vi "3.7-Reliable UDP Server Template.vi"() -> ()   [LabVIEW 2010]
doc: "UDP Mutlicast Addressing Scheme:\n\n3.7 - Multicast Address: 133.7.3.7\n3.1-4.7.1 Port: 31471\n3.2-4.7.2 Port: 32472\n3.3-4.7.3 Port: 33473\n3.4-4.7.4 Port: 34474\n\n5.7 - Multicast Address: 133.7.5.7\n5.1-4.7.1 Port: 51471\n5.2-4.7.2 Port: 52472\n5.3-4.7.3 Port: 53473\n5.4-4.7.4 Port: 54474\n\n5.1-6.7.1 Port: 51671\n5.2-6.7.2 Port: 52672\n5.3-6.7.3 Port: 53673\n5.4-6.7.4 Port: 54674\n\n7.7 - Multicast Address: 133.7.7.7\n7.1-6.7.1 Port: 61671\n7.2-6.7.2 Port: 62672\n7.3-6.7.3 Port: 63673\n7.4-6.7.4 Port: 64674"
uses:
  4-High Neurons/4.0-Super Heart Beat.ctl
  <vilib>/Utility/tcp.llb/UDP Multicast Write-Only Open.vi
  3.0-Global.vi
panel:
  out "Error":errorcluster
  in  "stop":bool
  out "Super Heart Beat":T1
  out "Processed":string
  in  "Debug Data":string
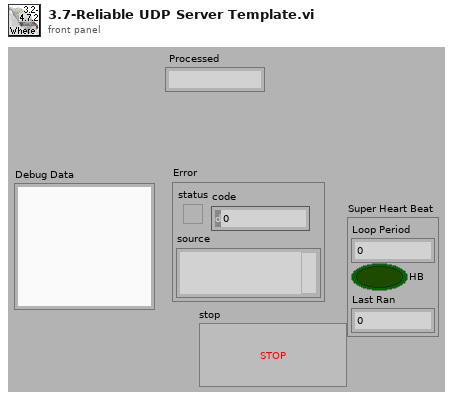
[diagram p1: front panel]
types:
  T1 = typedef "4.0-Super Heart Beat.ctl" = cluster{"Loop Period":u32, "HB":bool, "Last Ran":u32}
  T2 = typedef "3.3-What Sensor Typedef.ctl" = cluster{"LIDAR Data":T3}
  T3 = typedef "3.3.1-LIDAR Data Typedef.ctl" = cluster{"Angle array":dbl[], "Magnitude array ":dbl[]}
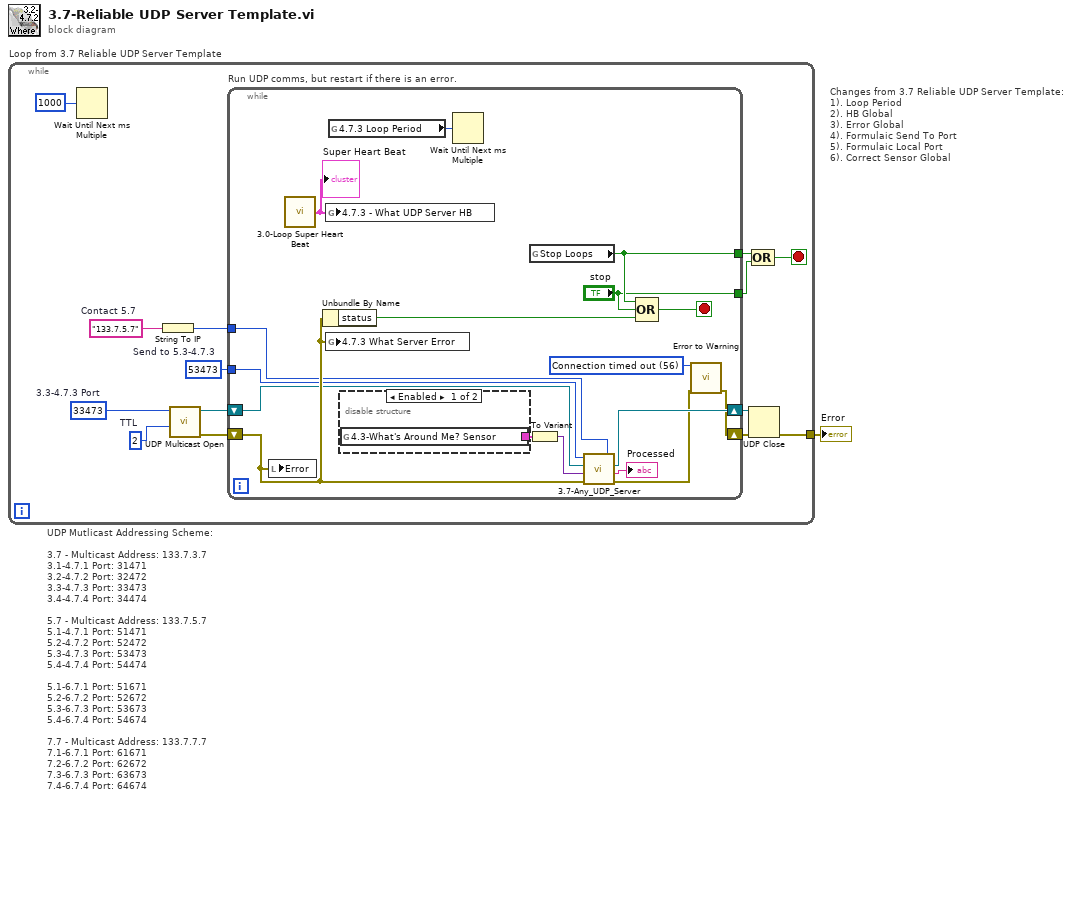
[diagram p0: block diagram]
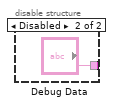
[diagram p2: hidden frame]
diagram:
  # "Changes from 3.7 Reliable UDP Server Template:\n1). Loop Period\n2). HB Global\n3). Error Global\n4). Formulaic Send To Port\n5). Formulaic Local Port\n6). Correct Sensor Global"
  # "UDP Mutlicast Addressing Scheme:\n\n3.7 - Multicast Address: 133.7.3.7\n3.1-4.7.1 Port: 31471\n3.2-4.7.2 Port: 32472\n3.3-4.7.3 Port: 33473\n3.4-4.7.4 Port: 34474\n\n5.7 - Multicast Address: 133.7.5.7\n5.1-4.7.1 Port: 51471\n5.2-4.7.2 Port: 52472\n5.3-4.7.3 Port: 53473\n5.4-4.7.4 Port: 54474\n\n5.1-6.7.1 Port: 51671\n5.2-6.7.2 Port: 52672\n5.3-6.7.3 Port: 53673\n5.4-6.7.4 Port: 54674\n\n7.7 - Multicast Address: 133.7.7.7\n7.1-6.7.1 Port: 61671\n7.2-6.7.2 Port: 62672\n7.3-6.7.3 Port: 63673\n7.4-6.7.4 Port: 64674"
  n1 = while "Loop from 3.7 Reliable UDP Server Template" {
    tunnel: [w10] -> w1
    stop <- w13 stop-if-true
    w2 = "133.7.5.7"  # Contact 5.7
    w4 = u16 53473  # Send to 5.3-4.7.3
    w7 = u16 2  # TTL
    w8 = u16 33473  # 3.3-4.7.3 Port
    n2 = Wait Until Next ms Multiple(millisecond multiple=u32 1000) -> ()  [unwired: 1 out]
    n3 = String To IP(1:w2) -> (0:w3:u32)
    n4 = call-poly <vilib>:"UDP Multicast Open.vi"("time-to-live (1)"=w7, "port"=w8) -> ("error out"=w5:errorcluster, "connection ID"=w6:refnum<k16>)  [unwired: 8 in]
    n5 = while "Run UDP comms, but restart if there is an error." {
      tunnel: [w31] -> w15
      tunnel: ["stop"] -> w14
      shift-right: [w22] -> w12
      shift-left: w6 -> [w23]
      shift-right: [w17] -> w11
      shift-left: w5 -> [w27]
      tunnel: w4 -> [w21]
      tunnel: w3 -> [w20]
      stop <- w32 stop-if-true
      w18 = 56 items=["No Error", "Argument Error", "Memory Full", "Out of Zone", "End of File", "File Already Open", "Generic File IO Error", "File Not Found", "File Permission Error", "Disk Full", "Duplicate Path", "Too Many Files Open", "Not Enabled", "Resource File Not Found", "Cannot Add Resource", "Resource Not Found", "Image Not Found", "Image Memory Error", "Pen Does Not Exist", "Config Bad Type", "Config Token Not Found", "Config Parse Error", "Config Memory Error", "Bad External Code Format", "Bad External Code Offset", "External Code Not Present", "Null Window", "Destroy Window Mixup", "Null Menu", "Print Aborted", "Bad Print Record", "Print Driver Error", "Windows Error During Print", "Memory Error During Print", "Print Dialog Error", "Generic Print Error", "Invalid Device Refnum", "Device Not Found", "Device Parameter Error", "Device Unit Error", "Can't Open Device", "Device Call Aborted", "Generic Error", "Cancelled By User", "Object ID Too Low", "Object ID Too High", "Object Not In Heap", "Unknown Heap", "Bad DefProc ID", "DefProc Not In Table", "Message Out Of Range", "Null Method", "Unknown Message", "Manager Call Not Supported", "Bad address", "Connection In progress", "Connection timed out", "Connection is already in progress", "Network attribute not supported", "Network error", "Address in use", "System out of memory", "Connection aborted", "Connection refused", "Connection is not connected", "Connection is already connected", "Connection closed", "Initialize error (interapplication manager)", "Bad occurrence", "Wait on unbound occurrence handler", "Occurrence queue overflow", "Bad path", "Semaphore not signaled", "Unrecognized type (interapplication manager)"] ("1st Error to Convert")
      n6 = local write "Error"(w27) -> ()
      n7 = call "3.0-Loop Super Heart Beat.vi"() -> ("Super Heart Beat"=w26:T1)
      "Super Heart Beat" <- w26
      n8 = Unbundle By Name(w27) -> ("status"=w29:bool)
      n9 = global write "3.0-Global.vi" "4.7.3 - What UDP Server HB"(w26) -> ()
      n10 = global write "3.0-Global.vi" "4.7.3 What Server Error"(w27) -> ()
      n11 = global read "3.0-Global.vi" "4.7.3 Loop Period"() -> (w16:u32)
      n12 = disable-structure shown="Enabled" {
        disable-tunnel: [w33 "Debug Data"] -> w25
        frame Enabled {
          n13 = global read "3.0-Global.vi" "4.3-What's Around Me? Sensor"() -> (w33:T2)
        }
        frame Disabled {
        }
      }
      n14 = Wait Until Next ms Multiple(millisecond multiple=w16) -> ()  [unwired: 1 out]
      n15 = global read "3.0-Global.vi" "Stop Loops"() -> (w31:bool)
      n16 = To Variant(anything=w25) -> (Variant=w28:variant)
      n17 = call "3.7-Any_UDP_Server.vi"("Multicast Address"=w20, "error In"=w27, "Data in"=w28, "Connection ID"=w23, "Send To Port"=w21) -> ("warning out"=w19:errorcluster, "Processed"=→"Processed":string, "Connection ID out"=w22:refnum<k16>)
      n18 = Compound Arithmetic op=OR(w31, "stop", w29) -> (w32:bool)
      n19 = call <vilib>:"Error to Warning.vi"("1st Error to Convert"=w18, "error in"=w19) -> ("warning out"=w17:errorcluster)  [unwired: 13 in]
    }
    n20 = UDP Close(connection ID=w12, 8:w11) -> (error out=w10:errorcluster)  [unwired: 1 out]
    n21 = Compound Arithmetic op=OR(w15, w14) -> (w13:bool)
  }
  "Error" <- w1
